vi "subVI_PID.vi"(8 "Cumulative Error In":dbl, 9 "Previous Error":dbl, 10 "Encoder Position [mm]":dbl, 11 "Desired Position [mm]":dbl) -> (0 "Cumulative Error Out":dbl, 1 "Error":dbl, 3 "Control Signal [V]":dbl)   [LabVIEW 2019]
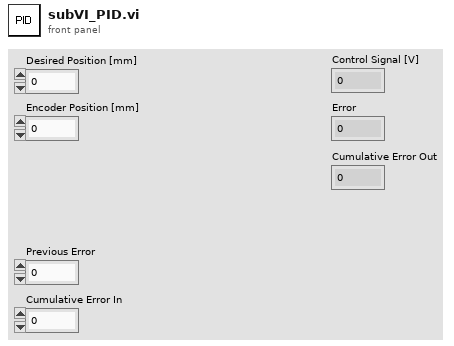
[diagram p1: front panel]
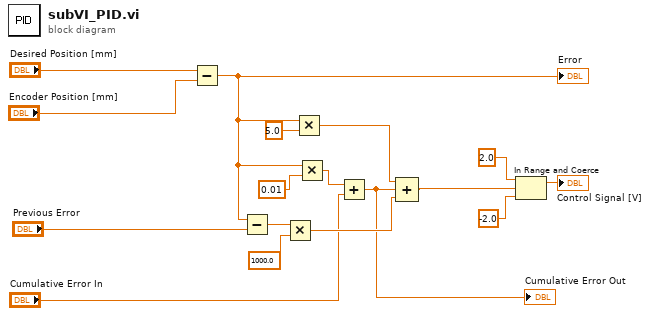
[diagram p0: block diagram]
diagram:
  n1 = Subtract(x="Desired Position [mm]", y="Encoder Position [mm]") -> (x-y=w15:dbl)
  "Error" <- w15
  n2 = Subtract(x=w15, y="Previous Error") -> (x-y=w13:dbl)
  n3 = Multiply(x=w13, y=1000.0) -> (x*y=w11:dbl)
  n4 = Multiply(x=w15, y=5.0) -> (x*y=w12:dbl)
  n5 = Multiply(x=w15, y=0.01) -> (x*y=w9:dbl)
  n6 = Add(x=w9, y="Cumulative Error In") -> (x+y=w5:dbl)
  "Cumulative Error Out" <- w5
  n7 = Compound Arithmetic op=ADD(w12, w5, w11) -> (w1:dbl)
  n8 = In Range and Coerce(upper limit=2.0, x=w1, lower limit=-2.0) -> (coerced(x)=→"Control Signal [V]":dbl)  [unwired: 1 out]
